vi "Get Tagged Packet Offsets.vi"(0 "tdms file in":refnum<k34>, 11 "error in":errorcluster) -> (4 "tdms file out":refnum<k34>, 6 "tagged packet offsets":i64[](array[numeric]), 8 "packet offsets valid?":bool, 15 "error out":errorcluster)   [LabVIEW 2023, in "GettingStarted_Common_148X_Host.lvlib"]
uses:
  GettingStarted_Common_148X_Host.lvlib
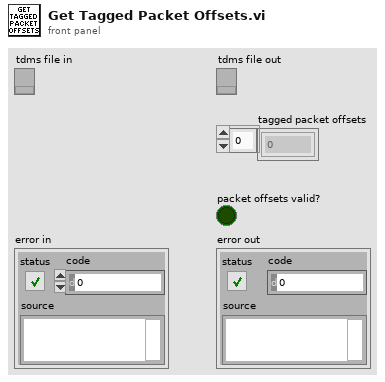
[diagram p1: front panel]
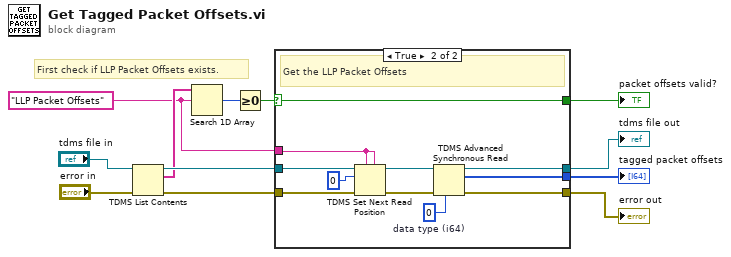
[diagram p0: block diagram]
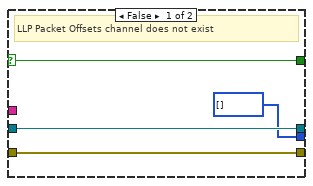
[diagram p2: hidden frame]
diagram:
  w5 = "LLP Packet Offsets" ("channel and group name")
  # "First check if LLP Packet Offsets exists."
  n1 = TDMS List Contents(4:"error in", 7:"tdms file in") -> (0:w9:errorcluster, 2:w6:string[], 3:w10:refnum<k34>)  [unwired: 1 in, 1 out]
  n2 = Search 1D Array(1D array=w6, element=w5) -> (index of element=w4:i32)  [unwired: 1 in]
  n3 = Greater Or Equal To 0?(x=w4) -> (x >= 0?=w3:bool)
  n4 = case shown="True" w3 {
    selector: w3 -> [w14 w20]
    tunnel: w10 -> [w15 w23]
    tunnel: w9 -> [w16 w22]
    tunnel: w5 -> [_ w21]
    tunnel: [w16 w18] -> w8
    tunnel: [w15 w19] -> w7
    tunnel: [w14 w20] -> w2
    tunnel: [i64[] [] w17] -> w1
    frame False {
      # "LLP Packet Offsets channel does not exist"
    }
    frame True {
      w24 = i64 0  # data type (i64)
      # "Get the LLP Packet Offsets"
      n5 = TDMS Set Next Read Position(5:w21, 7:w21, 8:w22, 10:i64 0 ("offset (0)"), 11:w23) -> (0:w25:errorcluster, 3:w26:refnum<k34>)  [unwired: 1 in]
      n6 = TDMS Advanced Synchronous Read(6:w24, 8:w25, 11:w26) -> (0:w18:errorcluster, 2:w17:i64[], 3:w19:refnum<k34>)  [unwired: 1 in, 1 out]
    }
  }
  "error out" <- w8
  "tdms file out" <- w7
  "packet offsets valid?" <- w2
  "tagged packet offsets" <- w1
